vi "RTS Chamber Control CMD.vi"(8 "Error In":errorcluster, 11 "Room Setpoints":T1={"Room Setpoint Temperature (*RM Dry Set P1)"=90.0, "Room Setpoint Humidity (*RM Hum Set P1)"=20.0, "Room Cool Temperature (*RM Cool Setp 1)"=65.0, "Room Dehum Temperature (*RM De Hum Set P1)"=60.0} {"Room Dehum Temperature (*RM De Hum Set P1)" min=30.0 max=120.0; "Room Cool Temperature (*RM Cool Setp 1)" min=30.0 max=120.0; "Room Setpoint Humidity (*RM Hum Set P1)" min=5.0 max=98.0; "Room Setpoint Temperature (*RM Dry Set P1)" min=40.0 max=120.0}) -> (0 "Error Out":errorcluster, 3 "Output Command":string)   [LabVIEW 2016]
uses:
  Type Definitions/RTS Chamber Temperature Humidity Control.ctl
  Drivers/WAGO 750-881/Type Definitions/Wago Input Commands.ctl
  Type Definitions/RTS Custom Commands.ctl
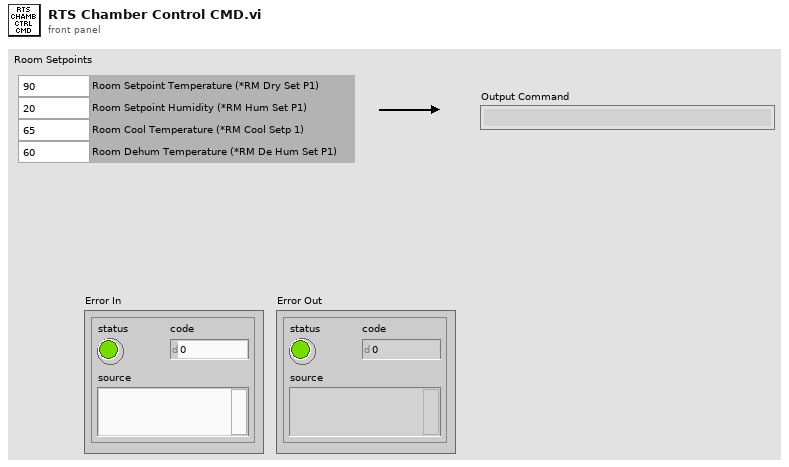
[diagram p1: front panel]
types:
  T1 = typedef "RTS Chamber Temperature Humidity Control.ctl" = cluster{"Room Setpoint Temperature (*RM Dry Set P1)":dbl, "Room Setpoint Humidity (*RM Hum Set P1)":dbl, "Room Cool Temperature (*RM Cool Setp 1)":dbl, "Room Dehum Temperature (*RM De Hum Set P1)":dbl}
  T2 = typedef "RTS Custom Commands.ctl" = string
  T3 = typedef "Wago Input Commands.ctl" = u16
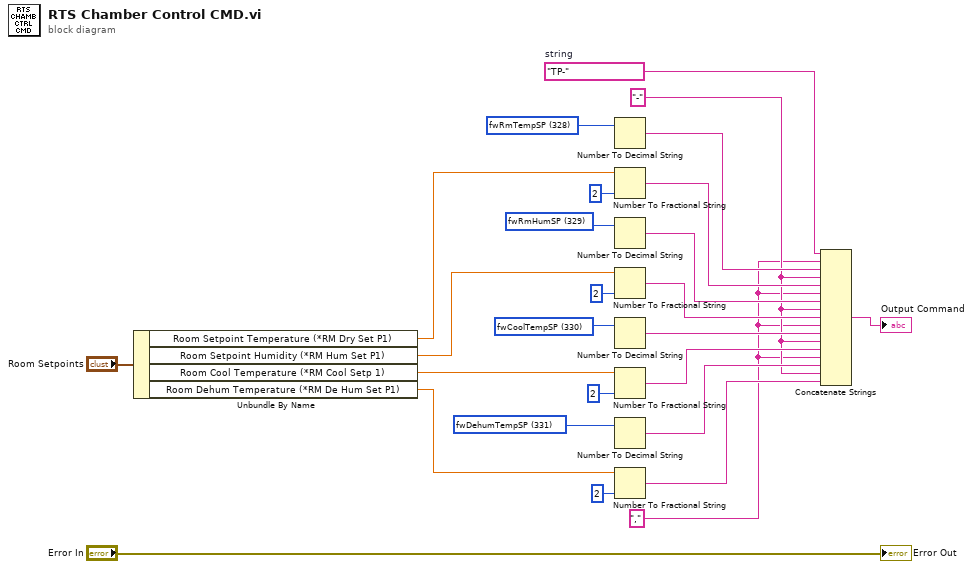
[diagram p0: block diagram]
diagram:
  w2 = T2 "TP-"  # string
  w3 = "-" ("string")
  w5 = T3 331 items=["fwS1Volt1"=0, "fwS1Volt2"=1, "fwS2Volt1"=2, "fwS2Volt2"=3, "fwS3Volt1"=4, "fwS3Volt2"=5, "fwS4Volt1"=6, "fwS4Volt2"=7, "fwS5Volt1"=8, "fwS5Volt2"=9, "fwS6Volt1"=10, "fwS6Volt2 "=11, "fwS7Volt1"=12, "fwS7Volt2"=13, "fwS8Volt1"=14, "fwS8Volt2"=15, "fwRoomHum"=16, "fwRoomTemp"=17, "fwAISpare1"=18, "fwAISpare2"=19, "fwSuppTemp"=20, "fwCoolTemp"=21, "fwDehumTemp"=22, "fwUnused"=23, "Bool Inputs"=24, "gwVoltRate1"=256, "gwVoltRate2"=257, "gwVoltRate3"=258, "gwVoltRate4"=259, "gwVoltRate5"=260, "gwVoltRate6"=261, "gwVoltRate7"=262, "gwVoltRate8"=263, "gwVoltWindow5/1"=264, "gwVoltWindow6/2"=265, "gwVoltWindow7/3"=266, "gwVoltWindow8/4"=267, "fwVoltSet1"=272, "fwVoltSet2"=273, "fwVoltSet3"=274, "fwVoltSet4"=275, "fwVoltSet5"=276, "fwVoltSet6"=277, "fwVoltSet7"=278, "fwVoltSet8"=279, "fwVoltRng1"=280, "fwVoltRng2"=281, "fwVoltRng3"=282, "fwVoltRng4"=283, "fwVoltRng5"=284, "fwVoltRng6"=285, "fwVoltRng7"=286, "fwVoltRng8"=287, "fwVoltPol1"=296, "fwVoltPol2"=297, "fwVoltPol3"=298, "fwVoltPol4"=299, "fwVoltPol5"=300, "fwVoltPol6"=301, "fwVoltPol7"=302, "fwVoltPol8"=303, "Rm1St1Dr1Cmd"=304, "Rm1St2Dr1Cmd"=305, "Rm1St3Dr1Cmd"=306, "Rm1St4Dr1Cmd"=307, "Rm1St5Dr1Cmd"=308, "Rm1St6Dr1Cmd"=309, "Rm1St7Dr1Cmd"=310, "Rm1St8Dr1Cmd"=311, "Rm1St1Dr2Cmd"=312, "Rm1St2Dr2Cmd"=313, "Rm1St3Dr2Cmd"=314, "Rm1St4Dr2Cmd"=315, "Rm1St5Dr2Cmd"=316, "Rm1St6Dr2Cmd"=317, "Rm1St7Dr2Cmd"=318, "Rm1St8Dr2Cmd"=319, "Rm1St1Dr3Cmd"=320, "Rm1St2Dr3Cmd"=321, "Rm1St3Dr3Cmd"=322, "Rm1St4Dr3Cmd"=323, "Rm1St5Dr3Cmd"=324, "Rm1St6Dr3Cmd"=325, "Rm1St7Dr3Cmd"=326, "Rm1St8Dr3Cmd"=327, "fwRmTempSP"=328, "fwRmHumSP"=329, "fwCoolTempSP"=330, "fwDehumTempSP"=331, "fwRmRun"=332, "fwRmOk"=333, "fwTesting"=334, "fwRmDryP"=335, "fwRmDryI"=336, "fwRmHumP"=337, "fwRmHumI"=338, "fwRmHeatP"=339, "fwRmHeatI"=340, "fwCoolTempP"=341, "fwCoolTempI"=342, "fwDehumTempP"=343, "fwDehumTempI"=344, "fwGndLeak1"=345, "fwGndLeak2"=346, "fwGndLeak3"=347, "fwGndLeak4"=348, "fwGndLeak5"=349, "fwGndLeak6"=350, "fwGndLeak7"=351, "fwGndLeak8"=352, "Rm1OpenerCmd"=353] ("Ring")
  w7 = T3 330 items=["fwS1Volt1"=0, "fwS1Volt2"=1, "fwS2Volt1"=2, "fwS2Volt2"=3, "fwS3Volt1"=4, "fwS3Volt2"=5, "fwS4Volt1"=6, "fwS4Volt2"=7, "fwS5Volt1"=8, "fwS5Volt2"=9, "fwS6Volt1"=10, "fwS6Volt2 "=11, "fwS7Volt1"=12, "fwS7Volt2"=13, "fwS8Volt1"=14, "fwS8Volt2"=15, "fwRoomHum"=16, "fwRoomTemp"=17, "fwAISpare1"=18, "fwAISpare2"=19, "fwSuppTemp"=20, "fwCoolTemp"=21, "fwDehumTemp"=22, "fwUnused"=23, "Bool Inputs"=24, "gwVoltRate1"=256, "gwVoltRate2"=257, "gwVoltRate3"=258, "gwVoltRate4"=259, "gwVoltRate5"=260, "gwVoltRate6"=261, "gwVoltRate7"=262, "gwVoltRate8"=263, "gwVoltWindow5/1"=264, "gwVoltWindow6/2"=265, "gwVoltWindow7/3"=266, "gwVoltWindow8/4"=267, "fwVoltSet1"=272, "fwVoltSet2"=273, "fwVoltSet3"=274, "fwVoltSet4"=275, "fwVoltSet5"=276, "fwVoltSet6"=277, "fwVoltSet7"=278, "fwVoltSet8"=279, "fwVoltRng1"=280, "fwVoltRng2"=281, "fwVoltRng3"=282, "fwVoltRng4"=283, "fwVoltRng5"=284, "fwVoltRng6"=285, "fwVoltRng7"=286, "fwVoltRng8"=287, "fwVoltPol1"=296, "fwVoltPol2"=297, "fwVoltPol3"=298, "fwVoltPol4"=299, "fwVoltPol5"=300, "fwVoltPol6"=301, "fwVoltPol7"=302, "fwVoltPol8"=303, "Rm1St1Dr1Cmd"=304, "Rm1St2Dr1Cmd"=305, "Rm1St3Dr1Cmd"=306, "Rm1St4Dr1Cmd"=307, "Rm1St5Dr1Cmd"=308, "Rm1St6Dr1Cmd"=309, "Rm1St7Dr1Cmd"=310, "Rm1St8Dr1Cmd"=311, "Rm1St1Dr2Cmd"=312, "Rm1St2Dr2Cmd"=313, "Rm1St3Dr2Cmd"=314, "Rm1St4Dr2Cmd"=315, "Rm1St5Dr2Cmd"=316, "Rm1St6Dr2Cmd"=317, "Rm1St7Dr2Cmd"=318, "Rm1St8Dr2Cmd"=319, "Rm1St1Dr3Cmd"=320, "Rm1St2Dr3Cmd"=321, "Rm1St3Dr3Cmd"=322, "Rm1St4Dr3Cmd"=323, "Rm1St5Dr3Cmd"=324, "Rm1St6Dr3Cmd"=325, "Rm1St7Dr3Cmd"=326, "Rm1St8Dr3Cmd"=327, "fwRmTempSP"=328, "fwRmHumSP"=329, "fwCoolTempSP"=330, "fwDehumTempSP"=331, "fwRmRun"=332, "fwRmOk"=333, "fwTesting"=334, "fwRmDryP"=335, "fwRmDryI"=336, "fwRmHumP"=337, "fwRmHumI"=338, "fwRmHeatP"=339, "fwRmHeatI"=340, "fwCoolTempP"=341, "fwCoolTempI"=342, "fwDehumTempP"=343, "fwDehumTempI"=344, "fwGndLeak1"=345, "fwGndLeak2"=346, "fwGndLeak3"=347, "fwGndLeak4"=348, "fwGndLeak5"=349, "fwGndLeak6"=350, "fwGndLeak7"=351, "fwGndLeak8"=352, "Rm1OpenerCmd"=353] ("Ring")
  w9 = T3 329 items=["fwS1Volt1"=0, "fwS1Volt2"=1, "fwS2Volt1"=2, "fwS2Volt2"=3, "fwS3Volt1"=4, "fwS3Volt2"=5, "fwS4Volt1"=6, "fwS4Volt2"=7, "fwS5Volt1"=8, "fwS5Volt2"=9, "fwS6Volt1"=10, "fwS6Volt2 "=11, "fwS7Volt1"=12, "fwS7Volt2"=13, "fwS8Volt1"=14, "fwS8Volt2"=15, "fwRoomHum"=16, "fwRoomTemp"=17, "fwAISpare1"=18, "fwAISpare2"=19, "fwSuppTemp"=20, "fwCoolTemp"=21, "fwDehumTemp"=22, "fwUnused"=23, "Bool Inputs"=24, "gwVoltRate1"=256, "gwVoltRate2"=257, "gwVoltRate3"=258, "gwVoltRate4"=259, "gwVoltRate5"=260, "gwVoltRate6"=261, "gwVoltRate7"=262, "gwVoltRate8"=263, "gwVoltWindow5/1"=264, "gwVoltWindow6/2"=265, "gwVoltWindow7/3"=266, "gwVoltWindow8/4"=267, "fwVoltSet1"=272, "fwVoltSet2"=273, "fwVoltSet3"=274, "fwVoltSet4"=275, "fwVoltSet5"=276, "fwVoltSet6"=277, "fwVoltSet7"=278, "fwVoltSet8"=279, "fwVoltRng1"=280, "fwVoltRng2"=281, "fwVoltRng3"=282, "fwVoltRng4"=283, "fwVoltRng5"=284, "fwVoltRng6"=285, "fwVoltRng7"=286, "fwVoltRng8"=287, "fwVoltPol1"=296, "fwVoltPol2"=297, "fwVoltPol3"=298, "fwVoltPol4"=299, "fwVoltPol5"=300, "fwVoltPol6"=301, "fwVoltPol7"=302, "fwVoltPol8"=303, "Rm1St1Dr1Cmd"=304, "Rm1St2Dr1Cmd"=305, "Rm1St3Dr1Cmd"=306, "Rm1St4Dr1Cmd"=307, "Rm1St5Dr1Cmd"=308, "Rm1St6Dr1Cmd"=309, "Rm1St7Dr1Cmd"=310, "Rm1St8Dr1Cmd"=311, "Rm1St1Dr2Cmd"=312, "Rm1St2Dr2Cmd"=313, "Rm1St3Dr2Cmd"=314, "Rm1St4Dr2Cmd"=315, "Rm1St5Dr2Cmd"=316, "Rm1St6Dr2Cmd"=317, "Rm1St7Dr2Cmd"=318, "Rm1St8Dr2Cmd"=319, "Rm1St1Dr3Cmd"=320, "Rm1St2Dr3Cmd"=321, "Rm1St3Dr3Cmd"=322, "Rm1St4Dr3Cmd"=323, "Rm1St5Dr3Cmd"=324, "Rm1St6Dr3Cmd"=325, "Rm1St7Dr3Cmd"=326, "Rm1St8Dr3Cmd"=327, "fwRmTempSP"=328, "fwRmHumSP"=329, "fwCoolTempSP"=330, "fwDehumTempSP"=331, "fwRmRun"=332, "fwRmOk"=333, "fwTesting"=334, "fwRmDryP"=335, "fwRmDryI"=336, "fwRmHumP"=337, "fwRmHumI"=338, "fwRmHeatP"=339, "fwRmHeatI"=340, "fwCoolTempP"=341, "fwCoolTempI"=342, "fwDehumTempP"=343, "fwDehumTempI"=344, "fwGndLeak1"=345, "fwGndLeak2"=346, "fwGndLeak3"=347, "fwGndLeak4"=348, "fwGndLeak5"=349, "fwGndLeak6"=350, "fwGndLeak7"=351, "fwGndLeak8"=352, "Rm1OpenerCmd"=353] ("Ring")
  w11 = T3 328 items=["fwS1Volt1"=0, "fwS1Volt2"=1, "fwS2Volt1"=2, "fwS2Volt2"=3, "fwS3Volt1"=4, "fwS3Volt2"=5, "fwS4Volt1"=6, "fwS4Volt2"=7, "fwS5Volt1"=8, "fwS5Volt2"=9, "fwS6Volt1"=10, "fwS6Volt2 "=11, "fwS7Volt1"=12, "fwS7Volt2"=13, "fwS8Volt1"=14, "fwS8Volt2"=15, "fwRoomHum"=16, "fwRoomTemp"=17, "fwAISpare1"=18, "fwAISpare2"=19, "fwSuppTemp"=20, "fwCoolTemp"=21, "fwDehumTemp"=22, "fwUnused"=23, "Bool Inputs"=24, "gwVoltRate1"=256, "gwVoltRate2"=257, "gwVoltRate3"=258, "gwVoltRate4"=259, "gwVoltRate5"=260, "gwVoltRate6"=261, "gwVoltRate7"=262, "gwVoltRate8"=263, "gwVoltWindow5/1"=264, "gwVoltWindow6/2"=265, "gwVoltWindow7/3"=266, "gwVoltWindow8/4"=267, "fwVoltSet1"=272, "fwVoltSet2"=273, "fwVoltSet3"=274, "fwVoltSet4"=275, "fwVoltSet5"=276, "fwVoltSet6"=277, "fwVoltSet7"=278, "fwVoltSet8"=279, "fwVoltRng1"=280, "fwVoltRng2"=281, "fwVoltRng3"=282, "fwVoltRng4"=283, "fwVoltRng5"=284, "fwVoltRng6"=285, "fwVoltRng7"=286, "fwVoltRng8"=287, "fwVoltPol1"=296, "fwVoltPol2"=297, "fwVoltPol3"=298, "fwVoltPol4"=299, "fwVoltPol5"=300, "fwVoltPol6"=301, "fwVoltPol7"=302, "fwVoltPol8"=303, "Rm1St1Dr1Cmd"=304, "Rm1St2Dr1Cmd"=305, "Rm1St3Dr1Cmd"=306, "Rm1St4Dr1Cmd"=307, "Rm1St5Dr1Cmd"=308, "Rm1St6Dr1Cmd"=309, "Rm1St7Dr1Cmd"=310, "Rm1St8Dr1Cmd"=311, "Rm1St1Dr2Cmd"=312, "Rm1St2Dr2Cmd"=313, "Rm1St3Dr2Cmd"=314, "Rm1St4Dr2Cmd"=315, "Rm1St5Dr2Cmd"=316, "Rm1St6Dr2Cmd"=317, "Rm1St7Dr2Cmd"=318, "Rm1St8Dr2Cmd"=319, "Rm1St1Dr3Cmd"=320, "Rm1St2Dr3Cmd"=321, "Rm1St3Dr3Cmd"=322, "Rm1St4Dr3Cmd"=323, "Rm1St5Dr3Cmd"=324, "Rm1St6Dr3Cmd"=325, "Rm1St7Dr3Cmd"=326, "Rm1St8Dr3Cmd"=327, "fwRmTempSP"=328, "fwRmHumSP"=329, "fwCoolTempSP"=330, "fwDehumTempSP"=331, "fwRmRun"=332, "fwRmOk"=333, "fwTesting"=334, "fwRmDryP"=335, "fwRmDryI"=336, "fwRmHumP"=337, "fwRmHumI"=338, "fwRmHeatP"=339, "fwRmHeatI"=340, "fwCoolTempP"=341, "fwCoolTempI"=342, "fwDehumTempP"=343, "fwDehumTempI"=344, "fwGndLeak1"=345, "fwGndLeak2"=346, "fwGndLeak3"=347, "fwGndLeak4"=348, "fwGndLeak5"=349, "fwGndLeak6"=350, "fwGndLeak7"=351, "fwGndLeak8"=352, "Rm1OpenerCmd"=353] ("Ring")
  w1 = "," ("string")
  n1 = Unbundle By Name("Room Setpoints") -> ("Room Setpoint Temperature (*RM Dry Set P1)"=w23:dbl, "Room Setpoint Humidity (*RM Hum Set P1)"=w21:dbl, "Room Cool Temperature (*RM Cool Setp 1)"=w19:dbl, "Room Dehum Temperature (*RM De Hum Set P1)"=w17:dbl)
  n2 = Number To Decimal String(number=w11) -> (decimal integer string=w10:string)  [unwired: 1 in]
  n3 = Number To Fractional String(number=w23, precision (6)=i16 2) -> (F-format string=w16:string)  [unwired: 2 in]
  n4 = Number To Decimal String(number=w9) -> (decimal integer string=w8:string)  [unwired: 1 in]
  n5 = Number To Fractional String(number=w21, precision (6)=i16 2) -> (F-format string=w15:string)  [unwired: 2 in]
  n6 = Number To Decimal String(number=w7) -> (decimal integer string=w6:string)  [unwired: 1 in]
  n7 = Number To Fractional String(number=w19, precision (6)=i16 2) -> (F-format string=w14:string)  [unwired: 2 in]
  n8 = Number To Decimal String(number=w5) -> (decimal integer string=w4:string)  [unwired: 1 in]
  n9 = Number To Fractional String(number=w17, precision (6)=i16 2) -> (F-format string=w13:string)  [unwired: 2 in]
  n10 = Concatenate Strings(w2, w1, w10, w3, w16, w1, w8, w3, w15, w1, w6, w3, w14, w1, w4, w3, w13) -> (→"Output Command":string)
  "Error Out" <- "Error In"
